vi "UVSock_PRJ_UPDATE_GROUP.vi"(7 "new files":path[](array[path]), 8 "error in (no error)":errorcluster, 9 "Group":string, 10 "Target":string="Build Spec Name", 11 "project files":path[](array[path])) -> (0 "error out":errorcluster, 3 "project files out":path[](array[path]))   [LabVIEW 2011]
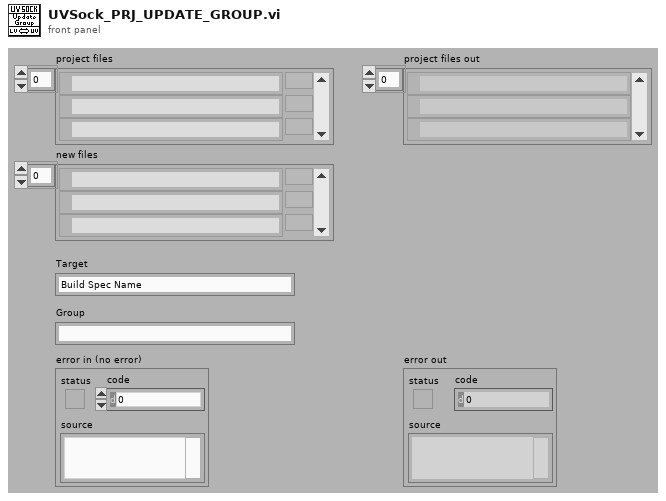
[diagram p1: front panel]
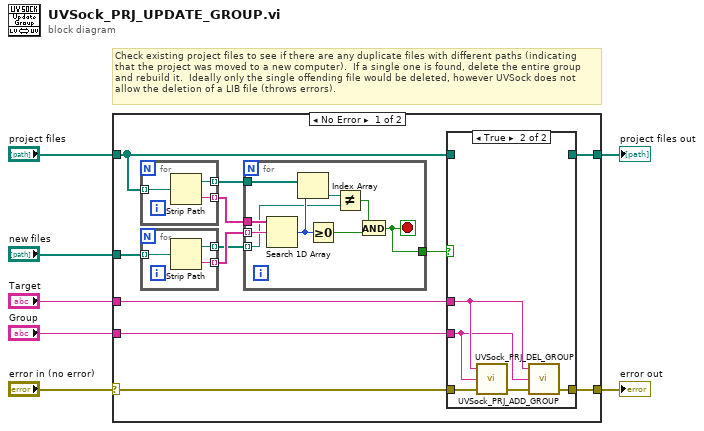
[diagram p0: block diagram]
diagram:
  # "Check existing project files to see if there are any duplicate files with different paths (indicating that the project was moved to a new computer).  If a single one is found, delete the entire group and rebuild it.  Ideally only the single offending file would be deleted, however UVSock does not allow the deletion of a LIB file (throws errors)."
  n1 = case shown="No Error" "error in (no error)" {
    selector: "error in (no error)" -> [w16 w43]
    tunnel: [w13 w43] -> w6
    tunnel: "project files" -> [w11 w42]
    tunnel: "new files" -> [w19 _]
    tunnel: "Target" -> [w15 _]
    tunnel: "Group" -> [w14 _]
    tunnel: [w10 w42] -> w1
    frame No Error {
      n2 = for {
        tunnel: [w41] -> w18 mode=indexing
        tunnel: w11 -> [w40] mode=indexing
        tunnel: [w39] -> w9 mode=indexing
        n3 = Strip Path(path=w40) -> (stripped path=w39:path, name=w41:string)
      }
      n4 = for {
        tunnel: [w38] -> w17 mode=indexing
        tunnel: w19 -> [w37] mode=indexing
        tunnel: [w36] -> w8 mode=indexing
        n5 = Strip Path(path=w37) -> (stripped path=w36:path, name=w38:string)
      }
      n6 = for {
        tunnel: w18 -> [w35]
        tunnel: w17 -> [w34] mode=indexing
        tunnel: [w27] -> w12
        tunnel: w9 -> [w32]
        tunnel: w8 -> [w30] mode=indexing
        stop <- w27 stop-if-true
        n7 = Search 1D Array(1D array=w35, element=w34) -> (index of element=w33:i32)  [unwired: 1 in]
        n8 = Index Array(array=w32, index=w33) -> (element=w31:path)
        n9 = Greater Or Equal To 0?(x=w33) -> (x >= 0?=w28:bool)
        n10 = Not Equal?(x=w31, y=w30) -> (x != y?=w29:bool)
        n11 = And(x=w29, y=w28) -> (x .and. y?=w27:bool)
      }
      n12 = case shown="True" w12 {
        tunnel: w16 -> [w21 w26]
        tunnel: w15 -> [_ w24]
        tunnel: w14 -> [_ w23]
        tunnel: [w21 w22] -> w13
        tunnel: w11 -> [w20 _]
        tunnel: [w20 _] -> w10
        frame False {
        }
        frame True {
          n13 = call "UVSock_PRJ_DEL_GROUP.vi"("error in (no error)"=w26, "Group"=w23, "Target"=w24) -> ("error out"=w25:errorcluster)  [unwired: 2 in]
          n14 = call "UVSock_PRJ_ADD_GROUP.vi"("error in (no error)"=w25, "Group"=w23, "Target"=w24) -> ("error out"=w22:errorcluster)  [unwired: 2 in]
        }
      }
    }
    frame Error {
    }
  }
  "project files out" <- w1
  "error out" <- w6
